vi "test_PinGroup_ReserveSessions_ChannelMappingsContainsAllPinsFromPinGroup.vi"() -> (6 "pass":bool, 8 "result":string, 15 "error out":errorcluster)   [LabVIEW 2020, in "MeasurementServerTests.lvlib" / "Session Reservation Tests.lvlib"]
uses:
  Session Reservation Tests.lvlib
  gRPC/Generated APIs/ni/measurementlink/sessionmanagement/v1/RPC Messages/ni_measurementlink_PinMapContext.ctl
  gRPC/Generated APIs/ni/measurementlink/sessionmanagement/v1/ni.measurementlink.sessionmanagement.v1.lvlib
  gRPC/Generated APIs/ni/measurementlink/sessionmanagement/v1/RPC Messages/ni_measurementlink_sessionmanagement_v1_ChannelMapping.ctl
  gRPC/Generated APIs/ni/measurementlink/sessionmanagement/v1/RPC Messages/nidevice_grpc_Session.ctl
  gRPC/Generated APIs/ni/measurementlink/sessionmanagement/v1/RPC Messages/ni_measurementlink_sessionmanagement_v1_SessionInformation.ctl
  3347d1b6-dca7-4e1a-9ca0-c9ec2f5aba95.vi
  ab61e54b-70f9-4719-86d2-c3025959eeb5.vi
  MeasurementServerTests.lvlib
  Runtime/APIs/Session Management V1/Session Reservation/Session Reservation.lvclass
panel:
  # "Test assumes discovery service, pin map service, and session management service have already been started."
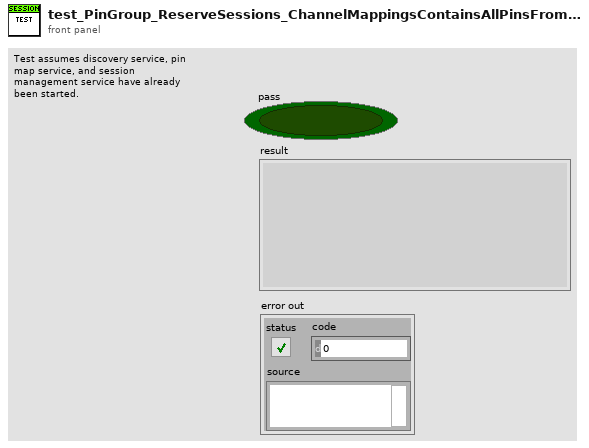
[diagram p1: front panel]
types:
  T1 = typedef "ni.measurementlink.sessionmanagement.v1.lvlib/ni_measurementlink_sessionmanagement_v1_SessionInformation.ctl" = cluster{"session":T2, "resource_name":string, "channel_list":string, "instrument_type_id":string, "session_exists":bool, "channel_mappings":T3[]}
  T2 = typedef "ni.measurementlink.sessionmanagement.v1.lvlib/nidevice_grpc_Session.ctl" = cluster{"name":string}
  T3 = typedef "ni.measurementlink.sessionmanagement.v1.lvlib/ni_measurementlink_sessionmanagement_v1_ChannelMapping.ctl" = cluster{"pin_or_relay_name":string, "site":i32, "channel":string, "multiplexer_resource_name":string, "multiplexer_route":string}
  T4 = typedef "ni.measurementlink.sessionmanagement.v1.lvlib/ni_measurementlink_PinMapContext.ctl" = cluster{"pin_map_id":string, "sites":i32[]}
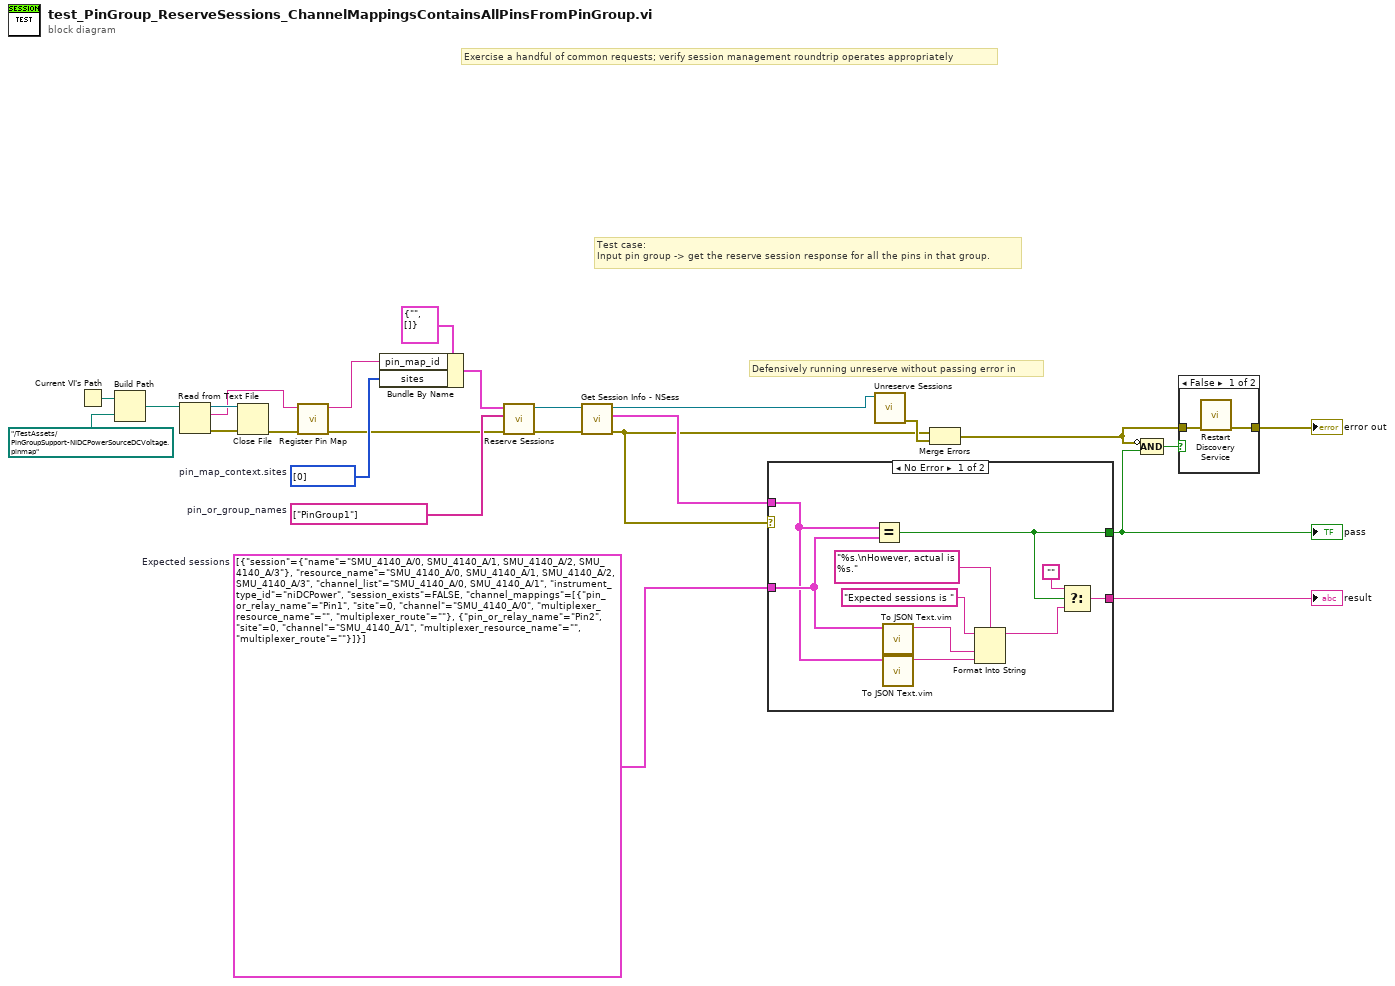
[diagram p0: block diagram]
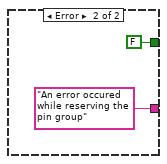
[diagram p2: hidden frame]
diagram:
  w14 = T1[] [{"session"={"name"="SMU_4140_A/0, SMU_4140_A/1, SMU_4140_A/2, SMU_4140_A/3"}, "resource_name"="SMU_4140_A/0, SMU_4140_A/1, SMU_4140_A/2, SMU_4140_A/3", "channel_list"="SMU_4140_A/0, SMU_4140_A/1", "instrument_type_id"="niDCPower", "session_exists"=FALSE, "channel_mappings"=[{"pin_or_relay_name"="Pin1", "site"=0, "channel"="SMU_4140_A/0", "multiplexer_resource_name"="", "multiplexer_route"=""}, {"pin_or_relay_name"="Pin2", "site"=0, "channel"="SMU_4140_A/1", "multiplexer_resource_name"="", "multiplexer_route"=""}]}]  # Expected sessions
  w11 = string[] ["PinGroup1"]  # pin_or_group_names
  w16 = i32[] [0]  # pin_map_context.sites
  # "Defensively running unreserve without passing error in"
  # "Test case:\nInput pin group -> get the reserve session response for all the pins in that group."
  # "Exercise a handful of common requests; verify session management roundtrip operates appropriately"
  n1 = Current VI's Path() -> (path=w25:path)
  n2 = Build Path(base path=w25, name or relative path=path "../TestAssets/PinGroupSupport-NIDCPowerSourceDCVoltage.pinmap") -> (appended path=w23:path)
  n3 = Read from Text File(file (use dialog)=w23) -> (refnum out=w21:refnum<file>, text=w17:string, error out=w22:errorcluster)  [unwired: 3 in, 1 out]
  n4 = Close File(refnum=w21, error in=w22) -> (error out=w15:errorcluster)  [unwired: 1 out]
  n5 = call "Register Pin Map.vi"("error in"=w15, "pin map xml"=w17) -> ("error out"=w10:errorcluster, "pin map id"=w18:string)  [unwired: 8 in]
  n6 = Bundle By Name(cluster=T4 {"pin_map_id"="", "sites"=[]} ("pin map context"), "pin_map_id"=w18, "sites"=w16) -> (w12:T4)
  n7 = call "Reserve Sessions.vi"("error in"=w10, "pin or relay names"=w11, "pin map context"=w12) -> ("error out"=w6:errorcluster, "session reservation out"=w8:refnum<class "Session Reservation.lvclass">)  [unwired: 7 in]
  n8 = call "Get Session Info - NSess .vi"("error in"=w6, "session reservation in"=w8) -> ("error out"=w4:errorcluster, "sessions info"=w7:T1[], "session reservation out"=w5:refnum<class "Session Reservation.lvclass">)  [unwired: 7 in]
  n9 = case shown="No Error" w4 {
    tunnel: [w35 FALSE] -> w2
    tunnel: [w34 "An error occured while reserving the pin group" ("String")] -> w20
    tunnel: w14 -> [w27 _]
    tunnel: w7 -> [w26 _]
    frame No Error {
      n10 = Equal?(x=w26, y=w27) -> (x = y?=w35:bool)
      n11 = call "To JSON Text.vim"("Anything"=w27) -> ("<JSON>"=w30:string)  [unwired: 9 in, 1 out]
      n12 = call "To JSON Text.vim"("Anything"=w26) -> ("<JSON>"=w29:string)  [unwired: 9 in, 1 out]
      n13 = Format Into String(format string="%s.\nHowever, actual is %s.", initial string="Expected sessions is ", w30, w29) -> (resulting string=w28:string)  [unwired: 1 in, 1 out]
      n14 = Select(t="", s=w35, f=w28) -> (s? t:f=w34:string)
    }
    frame Error {
    }
  }
  "pass" <- w2
  "result" <- w20
  n15 = call "Unreserve Sessions.vi"("session reservation in"=w5) -> ("error out"=w9:errorcluster)  [unwired: 10 in]
  n16 = Merge Errors(w4, w9) -> (w1:errorcluster)
  n17 = Compound Arithmetic op=AND(invert w1, w2) -> (w3:bool)
  n18 = case shown="False" w3 {
    tunnel: [w39 w40] -> w13
    tunnel: w1 -> [w38 w40]
    frame False {
      n19 = call "Restart Discovery Service.vi"("error in"=w38) -> ("error out"=w39:errorcluster)  [unwired: 10 in]
    }
    frame True {
    }
  }
  "error out" <- w13
